vi "CAN Get Value.vi"(7 "BufferLength":u32, 8 "error in (no error)":errorcluster caption="错误输入（无错误）", 9 "Buffer":u32, 10 "Parameter":u8, 11 "Channel":u8) -> (0 "error out":errorcluster caption="错误输出", 1 "Buffer out":u32, 2 "Parameter 2":u8, 3 "function return":u32)   [LabVIEW 2021]
doc: "TPCANStatus __stdcall CAN_GetValue(\n TPCANHandle Channel, \n TPCANParameter Parameter, \n void* Buffer, \n DWORD BufferLength);"
uses:
  PCANBasic.dll
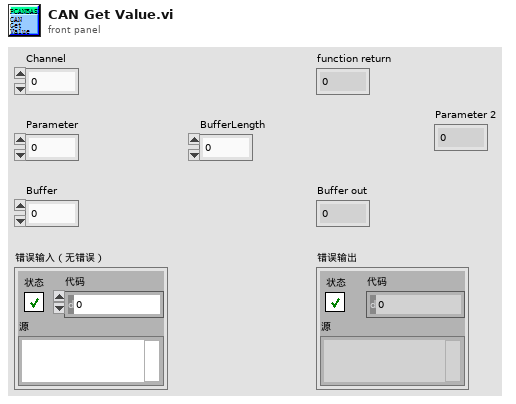
[diagram p1: front panel]
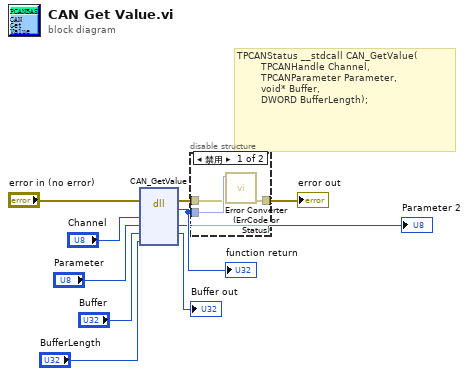
[diagram p0: block diagram]
diagram:
  # "TPCANStatus __stdcall CAN_GetValue(\n        TPCANHandle Channel, \n        TPCANParameter Parameter,  \n        void* Buffer, \n        DWORD BufferLength);"
  n1 = dll-call lib="D:/ON LINE WORK/LabVIEW/PCAN/PCAN 1.6(2021)/PCANBasic.*" fn="CAN_GetValue"(error in="error in (no error)", "Channel"="Channel", "Parameter"="Parameter", "Buffer"="Buffer", "BufferLength"="BufferLength") -> (error out=w5:errorcluster, "返回类型"=w10:u32, "Parameter"=→"Parameter 2":u8, "Buffer"=→"Buffer out":u32)  [unwired: 4 in, 1 out]
  "function return" <- w10
  n2 = disable-structure shown="禁用" {
    disable-tunnel: w10 -> [w13 _]
    disable-tunnel: w5 -> [w12 _]
    disable-tunnel: [w11 _] -> w4
    frame Disabled {
      n3 = call "Error Converter (ErrCode or Status).vi"("error in (no error)"=w12, "error code"=w13) -> ("error out"=w11:errorcluster)  [unwired: 9 in]
    }
    frame Enabled {
    }
  }
  "error out" <- w4
